vi "PostFlight Procedures.vi"() -> ()   [LabVIEW 2014]
panel:
  out "CO preflight Des 1":string="CO Monitor\n1.\tAL5002 plasma lamp\tturn off \t[front panel switch DWN]\n2.\tVacuum valve eV7 \t\tturn off\t[under AL5002 - CO tab]\n\n3.\tCOCYL1\t\t\tClose Manual Valves V1 & V2\t[clockwise]\n4.\tCOCYL2\t\t\tClose Manual Valves V3, V4 & V5\t[clockwise]\n5.\tCOCYL3\t\t\tClose cylinder valve\t\t\t[clockwise]\n6.\tNote down all CO cylinders content pressures [bottom gauge] at the end\n    of the flight in e-Log; compare with pre-flight values.  Pressure drops\n    should be maximum 10 bar.  Greater pressure drops are symptomatic of a\n    gas leak or ALREG pressure regulator failure.  Monitor pressure drop\n    carefully between flights or even in-flight if a leak is suspected.\n\n7.\tUPS\t\t\t\tSwitch off\t\t\t\t[down]\n\nUPS switch off should be BEFORE breaking 28Vdc CB, otherwise UPS battery will discharge itself.\n\n8.\t28Vdc\t\t\t\tBreak CB\n9.\t230Vac\t\t\tBreak CB\n\nFGGA \n10.\tFGGA Gas Stowage \tClose V1 and V3 on 3 gas cylinders;\nNote down content pressures in Core Chemistry e-Log\n\nSO2\nSO2 Span Gas\n11. Close cylinder valve 1 (clockwise).\n12. Close regulator valve 3 (clockwise).\n\nSO2 ZeroAir Gas\n13. Close cylinder valve 1 (clockwise).\n14. Back out (V2) delivery control valve (anticlockwise). \n\ne-Log\n11.\te-Log\t\t\t\tCopy/backup Bnnn_CoreChem_Log_v2.1 file onto Flight Manager's laptop Flights Folder if necessary.\n"
  in  "Exit":bool
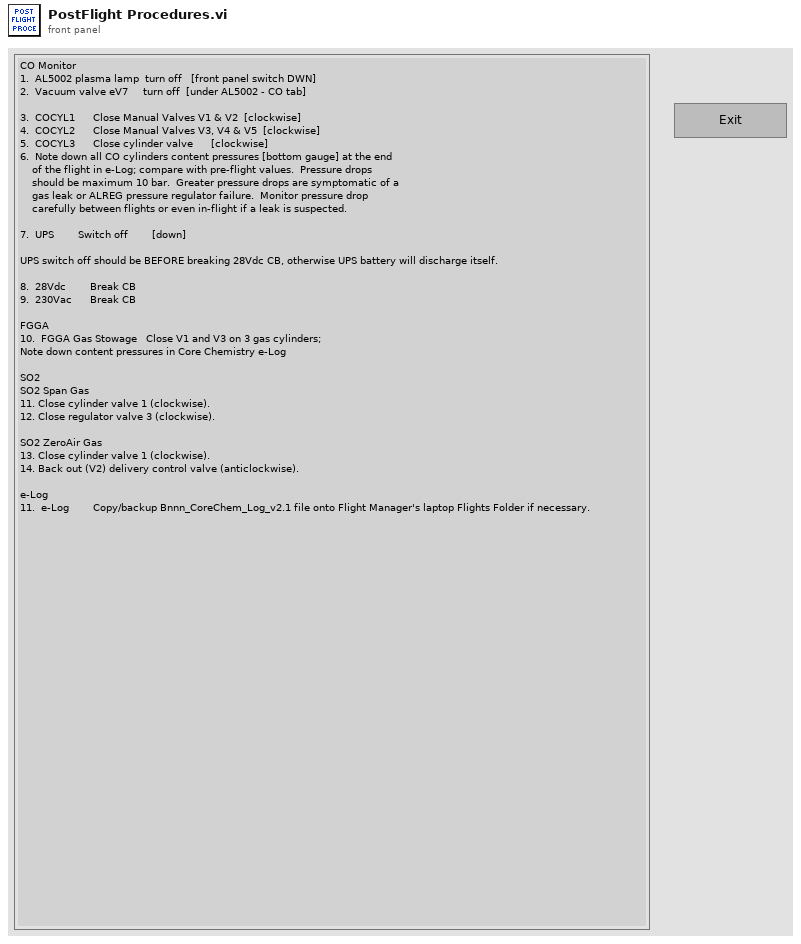
[diagram p1: front panel]
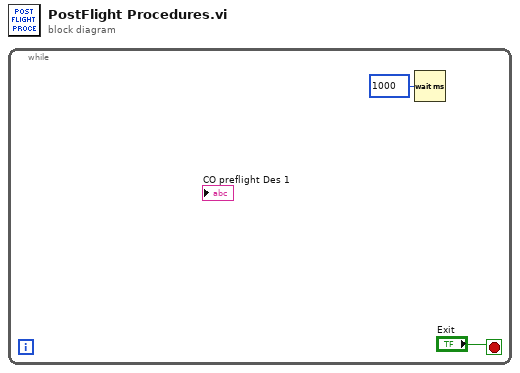
[diagram p0: block diagram]
diagram:
  n1 = while {
    stop <- "Exit" stop-if-true
    n2 = Wait (ms)(milliseconds to wait=u32 1000) -> ()  [unwired: 1 out]
  }
